vi "字符串匹配前两个字节山推.vi"(1 "匹配字节":string, 2 "待匹配字节":string) -> (0 "前两字节匹配与否":bool)   [LabVIEW 2016]
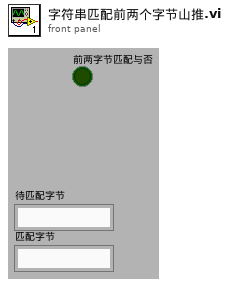
[diagram p1: front panel]
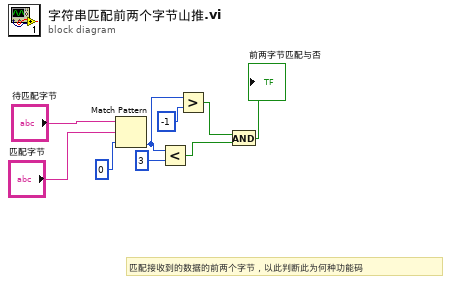
[diagram p0: block diagram]
diagram:
  # "匹配接收到的数据的前两个字节，以此判断此为何种功能码"
  n1 = Match Pattern(string="待匹配字节", regular expression="匹配字节", offset (0)=0 ("偏移量(0)")) -> (offset past match=w2:i32)  [unwired: 3 out]
  n2 = Less?(x=w2, y=3) -> (x < y?=w6:bool)
  n3 = Greater?(x=w2, y=-1) -> (0:w7:bool)
  n4 = And(x=w7, y=w6) -> (x .and. y?=→"前两字节匹配与否":bool)
